vi "Retrieve.vi"(8 "error in (no error)":errorcluster, 11 "Remote in":refnum<class "Remote.lvclass">) -> (0 "error out":errorcluster, 1 "Quem joga":string, 2 "Tabuleiro":T1, 3 "Remote out":refnum<class "Remote.lvclass">)   [LabVIEW 2017, in "Remote.lvclass"]
uses:
  Remote.lvclass
  controls/Tabuleiro.ctl
  Remote.lvclass/Remote.ctl
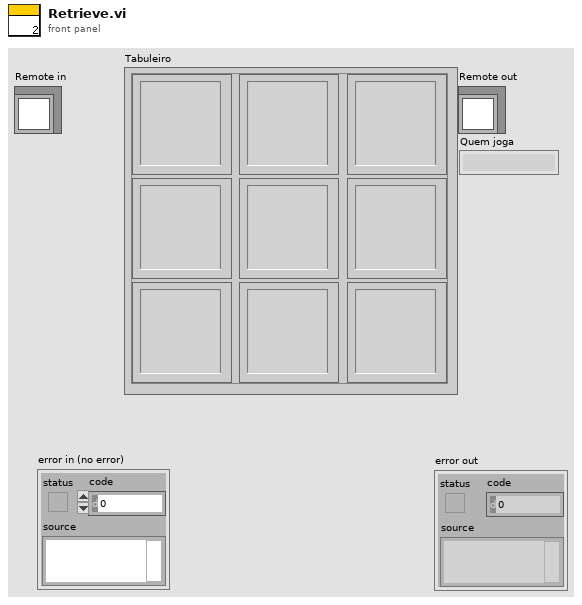
[diagram p1: front panel]
types:
  T1 = typedef "Tabuleiro.ctl" = cluster{"(0,0)":string, "(1,0)":string, "(0,1)":string, "(1,1)":string, "(2,0)":string, "(1,2)":string, "(2,2)":string, "(0,2)":string, "(2,1) ":string}
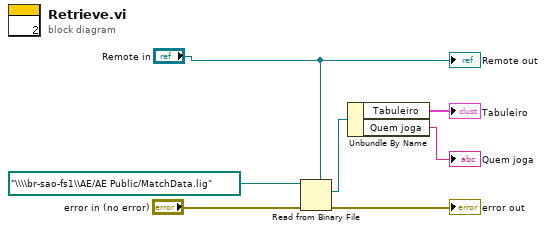
[diagram p0: block diagram]
diagram:
  n1 = Read from Binary File(5:"Remote in", 8:"error in (no error)", 11:path "\\\\br-sao-fs1\\AE/AE Public/MatchData.lig" ("file (use dialog)")) -> (0:→"error out":errorcluster, 2:w3:refnum<class "Remote.lvclass">)  [unwired: 3 in, 2 out]
  n2 = Unbundle By Name(w3) -> ("Tabuleiro"=→"Tabuleiro":T1, "Quem joga"=→"Quem joga":string)
  "Remote out" <- "Remote in"
